vi "Simulator.vi"(6 "error in (no error)":errorcluster, 8 "Distance Between Interpolated Points":dbl, 9 "Lithography Information":T1(array[cluster])) -> (0 "error out":errorcluster)   [LabVIEW 2011]
doc: "This VI controls the simulator."
uses:
  Global Variables.vi
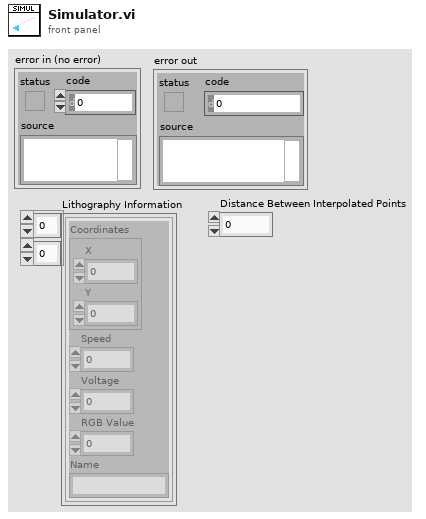
[diagram p1: front panel]
types:
  T1 = cluster{"Coordinates":cluster{"X":dbl, "Y":dbl}, "Speed":dbl, "Voltage":dbl, "RGB Value":i32, "Name":string}[][]
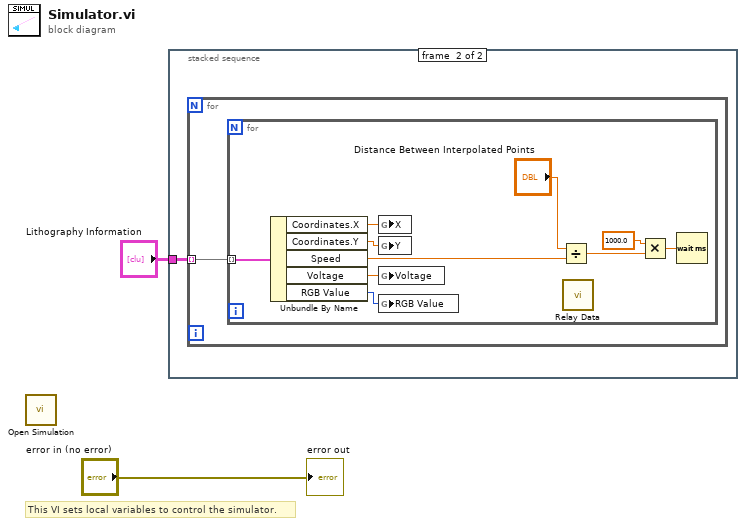
[diagram p0: block diagram]
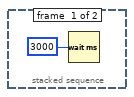
[diagram p2: hidden frame]
diagram:
  # "This VI sets local variables to control the simulator."
  n1 = call "Open Simulation.vi"() -> ()  [unwired: 12 in]
  n2 = stacked-sequence {
    tunnel: "Lithography Information" -> [_ w4]
    frame #0 {
      n3 = Wait (ms)(milliseconds to wait=u32 3000) -> ()  [unwired: 1 out]
    }
    frame #1 {
      n4 = for {
        tunnel: w4 -> [w5] mode=indexing
        n5 = for {
          tunnel: w5 -> [w13] mode=indexing
          n6 = Unbundle By Name(w13) -> ("Coordinates.X"=w14:dbl, "Coordinates.Y"=w15:dbl, "Speed"=w12:dbl, "Voltage"=w11:dbl, "RGB Value"=w10:i32)
          n7 = global write "Global Variables.vi" "X"(w14) -> ()
          n8 = global write "Global Variables.vi" "Y"(w15) -> ()
          n9 = global write "Global Variables.vi" "Voltage"(w11) -> ()
          n10 = global write "Global Variables.vi" "RGB Value"(w10) -> ()
          n11 = Divide(x="Distance Between Interpolated Points", y=w12) -> (x/y=w9:dbl)
          n12 = call "Relay Data.vi"() -> ()  [unwired: 12 in]
          n13 = Multiply(x=1000.0, y=w9) -> (x*y=w7:dbl)
          n14 = Wait (ms)(milliseconds to wait=w7) -> ()  [unwired: 1 out]
        }
      }
    }
  }
  "error out" <- "error in (no error)"
